vi "Post-Install Action.vi"() -> ()   [LabVIEW 2013]
uses:
  Types/Components Directory Install Files String Array.ctl
panel:
  out "Progress":u8(slide) scale=0.0..100.0
  out "TestStand Public Documents Directory":string="C:\\Users\\Public\\Documents\\National Instruments\\TestStand 2013\\Components\\TypePalettes"
  in  "OK Button":bool
  in  "Select TestStand Version to Install With:":u16(ring) items=["TestStand 2013", "TestStand 2014", "TestStand 2016"]
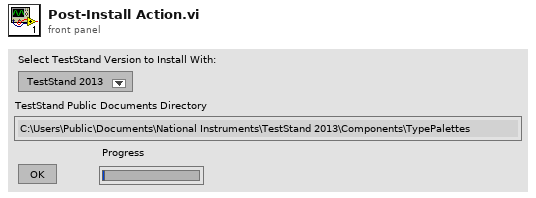
[diagram p1: front panel]
types:
  T1 = typedef "Components Directory Install Files String Array.ctl" = string[]
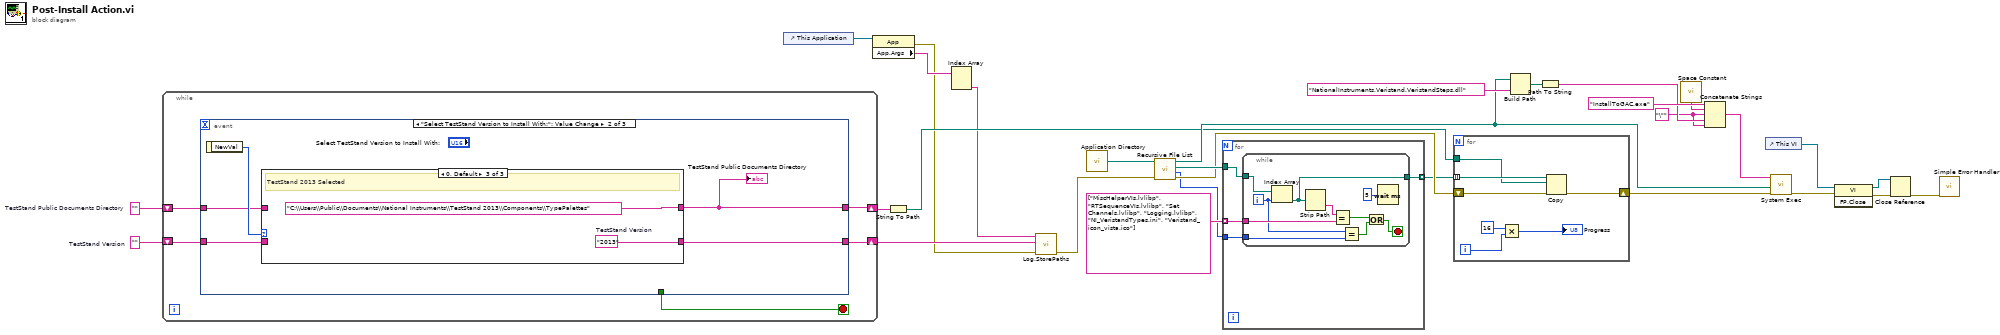
[diagram p0: block diagram]
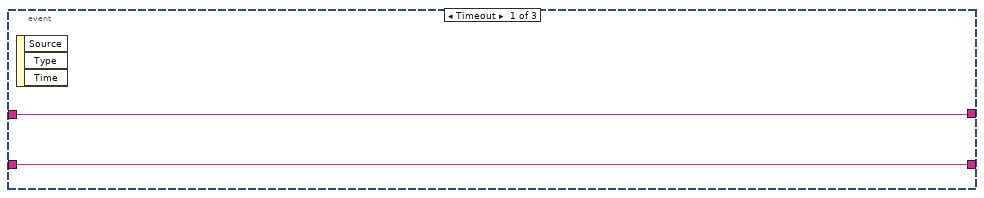
[diagram p2: hidden frame]
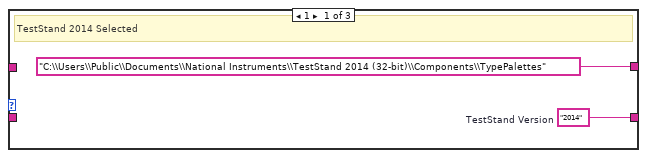
[diagram p3: hidden frame]
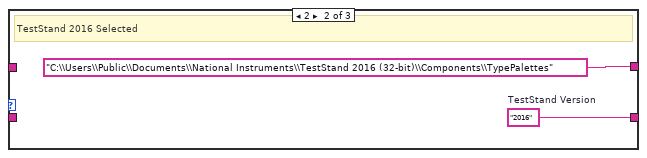
[diagram p4: hidden frame]
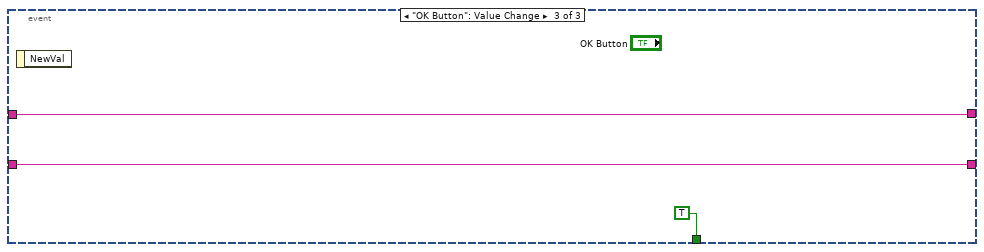
[diagram p5: hidden frame]
diagram:
  w5 = ""  # TestStand Version
  w8 = ""  # TestStand Public Documents Directory
  w12 = "\"" ("string")
  n1 = while {
    shift-right: [w34] -> w7
    shift-left: w8 -> [w35]
    shift-right: [w32] -> w4
    shift-left: w5 -> [w31]
    stop <- w33 stop-if-true
    n2 = event shown="[1] \"Select TestStand Version to Install With:\": Value Change" {
      selector: _ -> [_ _ _]
      dyn-events: _ -> [_ _ _]
      timeout: _ -> [_ _ _]
      tunnel: w35 -> [w37 w41 w50]
      tunnel: [w37 w40 w50] -> w34
      tunnel: [_ _ TRUE] -> w33
      tunnel: [w36 w39 w49] -> w32
      tunnel: w31 -> [w36 w38 w49]
      event Timeout {
        n3 = event-data() -> ()  [unwired: 1 in, 3 out]
      }
      event "Select TestStand Version to Install With:": Value Change {
        n4 = event-data() -> ("NewVal"=w42:u16)  [unwired: 1 in]
        n5 = case shown="0, Default" w42 {
          tunnel: w41 -> [_ _ _]
          tunnel: ["C:\\Users\\Public\\Documents\\National Instruments\\TestStand 2014 (32-bit)\\Components\\TypePalettes" ("TestStand Public Documents Directory") "C:\\Users\\Public\\Documents\\National Instruments\\TestStand 2016 (32-bit)\\Components\\TypePalettes" ("TestStand Public Documents Directory") "C:\\Users\\Public\\Documents\\National Instruments\\TestStand 2013\\Components\\TypePalettes" ("TestStand Public Documents Directory")] -> w40
          tunnel: [w43 w45 w47] -> w39
          tunnel: w38 -> [_ _ _]
          frame 1 {
            w43 = "2014"  # TestStand Version
            # "TestStand 2014 Selected"
          }
          frame 2 {
            w45 = "2016"  # TestStand Version
            # "TestStand 2016 Selected"
          }
          frame 0, Default {
            w47 = "2013"  # TestStand Version
            # "TestStand 2013 Selected"
          }
        }
        "TestStand Public Documents Directory" <- w40
      }
      event "OK Button": Value Change {
        n6 = event-data() -> ()  [unwired: 1 in, 1 out]
      }
    }
  }
  n7 = control-ref of="This Application"() -> (w9:refnum<vi>)
  n8 = property class="App"(reference=w9) -> (error out=w3:errorcluster, "App.Args"=w19:string[])  [unwired: 1 in, 1 out]
  n9 = String To Path(string=w7) -> (path=w6:path)
  n10 = Index Array(array=w19) -> (element #2=w2:string)  [unwired: 2 in, 1 out]
  n11 = call "Log.StorePaths.vi"("error in (no error)"=w3, "TestStand Version (2013)"=w4, "VeriStand Version (2013 SP1)"=w2) -> ("error out"=w1:errorcluster)  [unwired: 8 in]
  n12 = call <vilib>:"Application Directory.vi"() -> ("Application Directory"=w25:path)
  n13 = call <vilib>:"Recursive File List.vi"("error in (no error)"=w1, "Folder Path"=w25) -> ("error out"=w28:errorcluster, "Number of Files"=w27:i32, "All Files in Dir"=w30:path[], "dup Folder Path"=w10:path)  [unwired: 5 in, 1 out]
  n14 = for {
    tunnel: w30 -> [w54]
    tunnel: T1 ["MiscHelperVIs.lvlibp", "RTSequenceVIs.lvlibp", "Set Channels.lvlibp", "Logging.lvlibp", "NI_VeristandTypes.ini", "Veristand_icon_vista.ico"] -> [w55] mode=indexing
    tunnel: [w53] -> w26 mode=indexing
    tunnel: w27 -> [w52]
    n15 = while {
      tunnel: w55 -> [w64]
      tunnel: w54 -> [w63]
      tunnel: [w62] -> w53
      tunnel: w52 -> [w57]
      i -> [w59]
      stop <- w60 stop-if-true
      n16 = Index Array(array=w63, index=w59) -> (element=w62:path)
      n17 = Strip Path(path=w62) -> (name=w65:string)  [unwired: 1 out]
      n18 = Equal?(x=w65, y=w64) -> (x = y?=w61:bool)
      n19 = Equal?(x=w59, y=w57) -> (x = y?=w58:bool)
      n20 = Or(x=w61, y=w58) -> (x .or. y?=w60:bool)
      n21 = Wait (ms)(milliseconds to wait=u32 5) -> ()  [unwired: 1 out]
    }
  }
  n22 = for {
    tunnel: w26 -> [w71] mode=indexing
    shift-right: [w70] -> w24
    shift-left: w28 -> [w72]
    tunnel: w6 -> [w69]
    i -> [w67]
    n23 = Multiply(x=16, y=w67) -> (x*y=→"Progress":i32)
    n24 = Copy(8:w72, 10:w69, 11:w71) -> (0:w70:errorcluster)  [unwired: 2 in, 2 out]
  }
  n25 = Build Path(base path=w10, name or relative path="NationalInstruments.Veristand.VeristandSteps.dll" ("command line")) -> (appended path=w20:path)
  n26 = Path To String(path=w20) -> (string=w13:string)
  n27 = call <vilib>:"Space Constant.vi"() -> ("String"=w21:string)
  n28 = Concatenate Strings("InstallToGAC.exe" ("command line"), w21, w12, w13, w12) -> (w11:string)
  n29 = control-ref of="This VI"() -> (w18:refnum<vi>)
  n30 = call <vilib>:"System Exec.vi"("error in (no error)"=w24, "working directory"=w10, "command line"=w11) -> ("error out"=w14:errorcluster)  [unwired: 5 in, 3 out]
  n31 = invoke class="VI" method="FP.Close"(reference=w18, error in=w14) -> (reference out=w15:refnum<vi>, error out=w16:errorcluster)  [unwired: 1 in, 1 out]
  n32 = Close Reference(reference=w15, error in (no error)=w16) -> (error out=w17:errorcluster)
  n33 = call <vilib>:"Simple Error Handler.vi"("error in (no error)"=w17) -> ()  [unwired: 4 in, 5 out]
